vi "Main.vi"() -> ()   [LabVIEW 2021]
uses:
  Sub VIs/Trajectory Control/Trajectory_Control.ctl
  Sub VIs/Logging/Controller Data.ctl
  Sub VIs/Drive Motor/Drive Motor Data.ctl
  Sub VIs/Steering Motor/Steering Motor Data.ctl
  Sub VIs/State Estimator/State Estimate.ctl
  Sub VIs/State Estimator/Measurements.ctl
  Sub VIs/IMU/IMU Data.ctl
  Sub VIs/Steering Motor Encoder/Steering Motor Encoder Data.ctl
  Sub VIs/GNSS/GNSS Data.ctl
  <vilib>/Utility/RT CPU Load.ctl
  Sub VIs/Logging/Log Level.ctl
  <vilib>/Platform/TimedLoop/XDataNode/timing_clust.ctl
  <vilib>/Platform/TimedLoop/XDataNode/nitl_modes.ctl
  <vilib>/Platform/TimedLoop/XDataNode/wakeup.ctl
  Sub VIs/Steering Motor/Steering Motor Handle.ctl
  <vilib>/Platform/TimedLoop/XDataNode/XDataNode.xnode
  <vilib>/Platform/TimedLoop/XDataNode/XDNodeRunTimeDep.lvlib
  <vilib>/NI_Real-Time Target Support.lvlib
panel:
  in  "Abort Trajectory":bool
  in  "Kp":dbl
  in  "Ki":dbl
  out "Speed":bool
  in  "?":bool
  out "RPM":bool
  in  "Drive Motor Speed (m/s)":dbl
  in  "file path (trajectorymat)":path=path "c:/ni-rt/startup/trajectorymat_asta0_line.csv"
  in  "file path (matrixmat)":path=path "c:/ni-rt/startup/matrixmat_default.csv"
  out "velocity":dbl(graph)
  out "CPU loads":T1[](array[typedef]) {"ISR (%)" format="%#.2f"; "Idle (%)" format="%#.2f"; "Background (%)" format="%#.2f"; "Normal (%)" format="%#.2f"; "Above Normal (%)" format="%#.2f"; "High (%)" format="%#.2g"; "Timed Structures (%)" format="%#.2g"; "Time Critical (%)" format="%#.2g"; "Total (%)" format="%#.2g"}
  out "Measurements (Debug)":T2 {"GNSS Data"."Longitude (deg)" format="%#.10g"; "GNSS Data"."Latitude (deg)" format="%#.10g"; "GNSS Data"."Longitude (rad)" format="%#_10g"; "GNSS Data"."Latitude (rad)" format="%#_10g"}
  out "State Estimate (Debug)":T6 {"Y (m)" format="%#_10g"; "X (m)" format="%#_10g"}
  out "Motor Controllers (Debug)":T7
  out "Trajectory (Debug)":T10
  out "State estimator Ts check":bool
  out "E2 limit hit":bool
  out "E1 limit hit":bool
  out "XY trajectory (0 is bikeposition)":T11(graph)
  out "Y-Offset":dbl
  out "X-Offset":dbl
  in  "Reset and Init trajectory":bool
  in  "Drive Motor Angular Speed (rad/s)":dbl
  in  "Enable Steering Motor":bool
  out "Steering Motor Enabled":bool
  out "Abort":bool
  in  "Reset Steering Motor Encoder":bool
  in  "Stop Button":bool
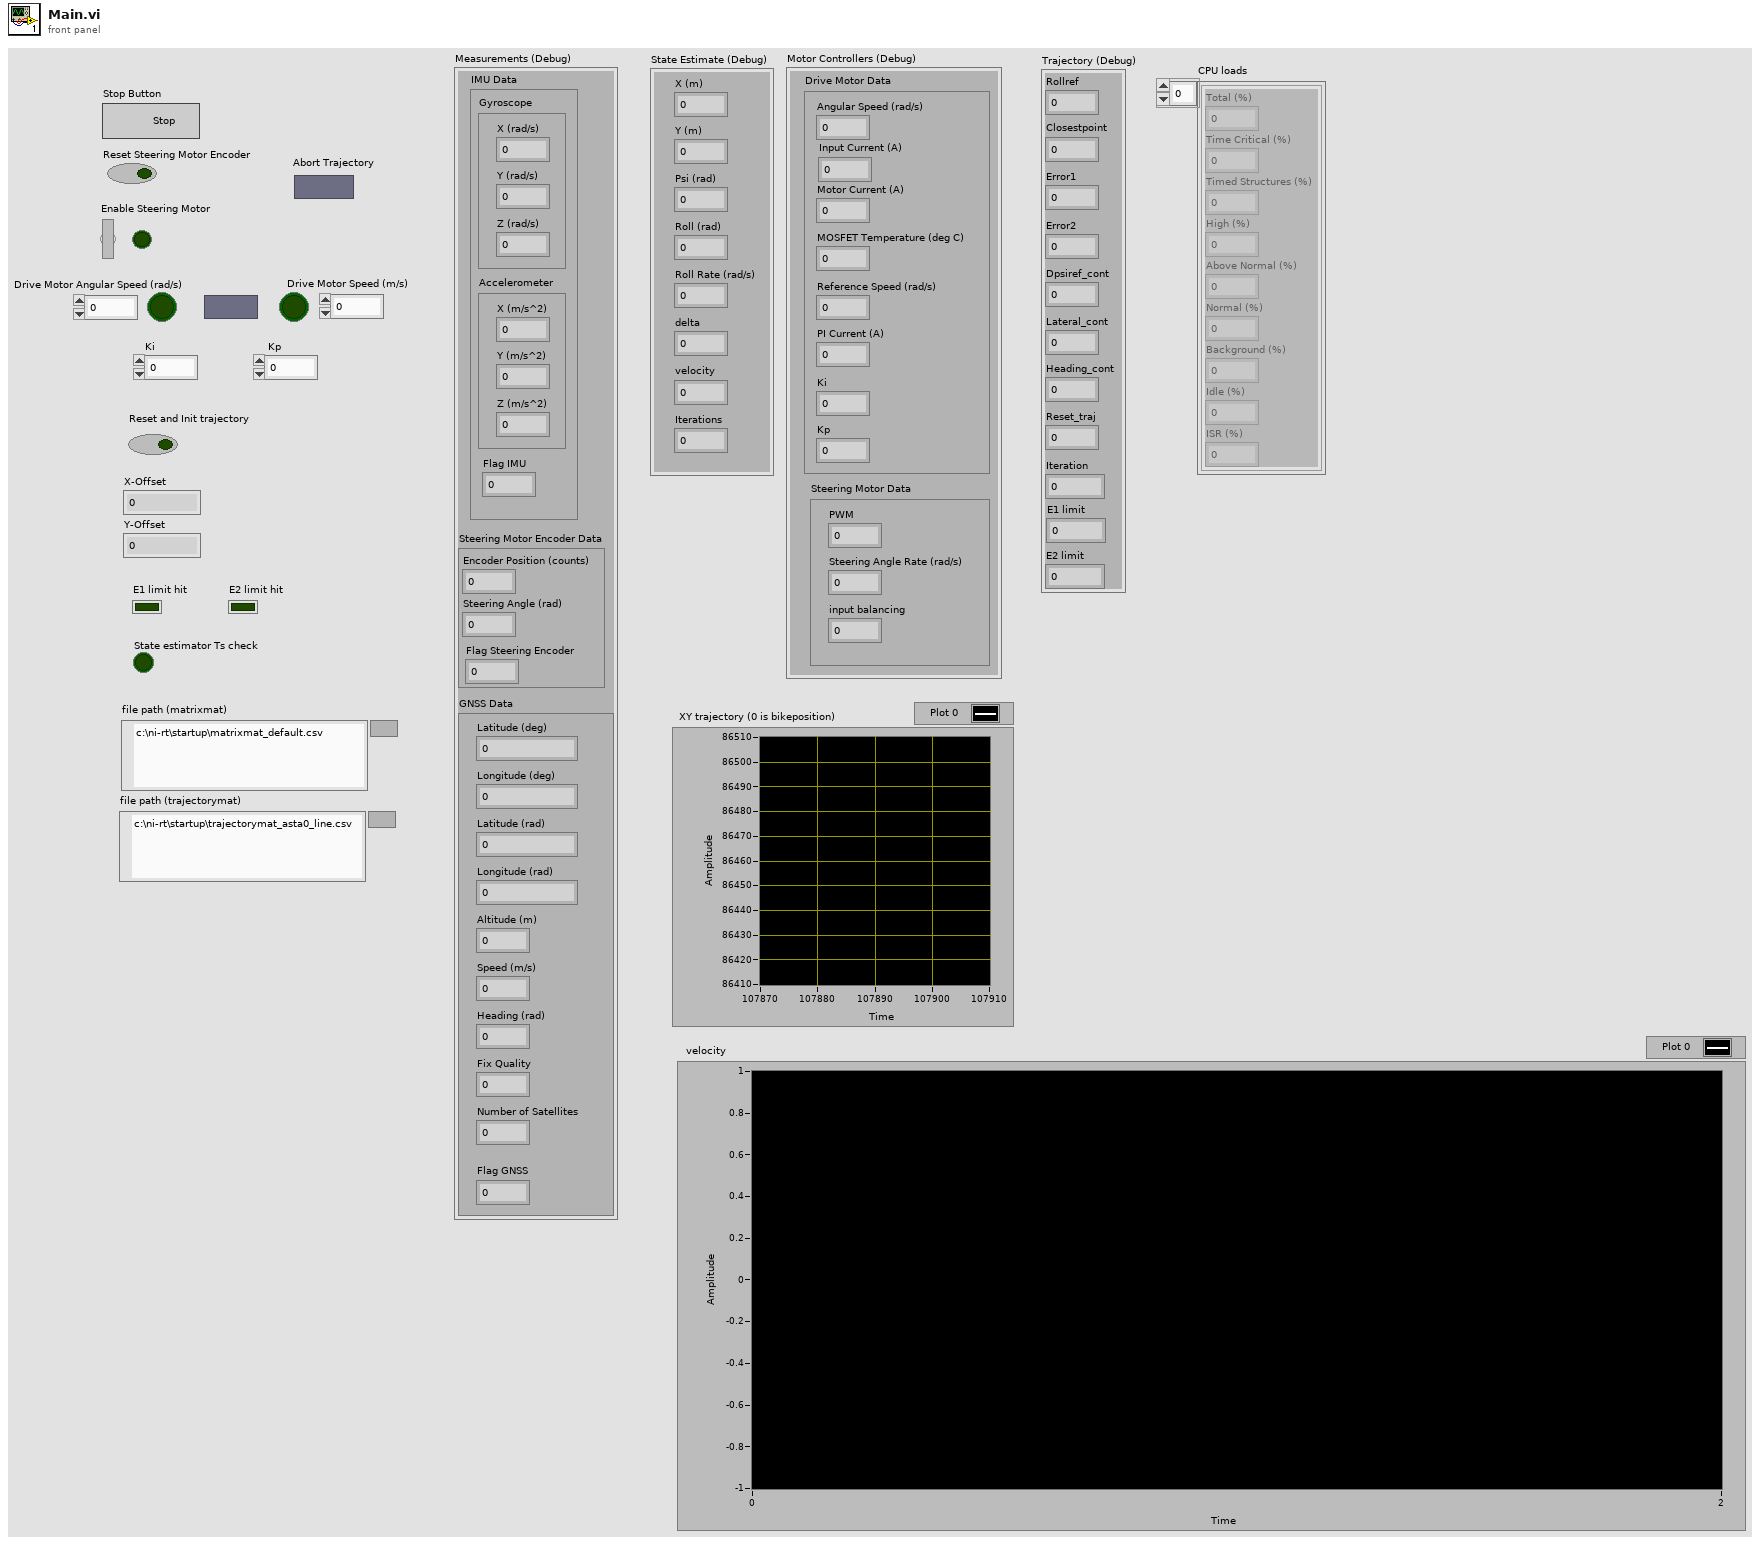
[diagram p1: front panel]
types:
  T1 = typedef "NI_Real-Time Target Support.lvlib/RT CPU Load.ctl" = cluster{"Total (%)":dbl, "Time Critical (%)":dbl, "Timed Structures (%)":dbl, "High (%)":dbl, "Above Normal (%)":dbl, "Normal (%)":dbl, "Background (%)":dbl, "Idle (%)":dbl, "ISR (%)":dbl}
  T2 = typedef "Measurements.ctl" = cluster{"IMU Data":T3, "Steering Motor Encoder Data":T4, "GNSS Data":T5}
  T3 = typedef "IMU Data.ctl" = cluster{"Gyroscope":cluster{"X (rad/s)":dbl, "Y (rad/s)":dbl, "Z (rad/s)":dbl}, "Accelerometer":cluster{"X (m/s^2)":dbl, "Y (m/s^2)":dbl, "Z (m/s^2)":dbl}, "Flag IMU":dbl}
  T4 = typedef "Steering Motor Encoder Data.ctl" = cluster{"Encoder Position (counts)":i32, "Steering Angle (rad)":dbl, "Flag Steering Encoder":dbl}
  T5 = typedef "GNSS Data.ctl" = cluster{"Latitude (rad)":dbl, "Longitude (rad)":dbl, "Altitude (m)":dbl, "Speed (m/s)":dbl, "Heading (rad)":dbl, "Fix Quality":i32, "Number of Satellites":i32, "Latitude (deg)":dbl, "Longitude (deg)":dbl, "Flag GNSS":dbl}
  T6 = typedef "State Estimate.ctl" = cluster{"X (m)":dbl, "Y (m)":dbl, "Psi (rad)":dbl, "Roll (rad)":dbl, "Roll Rate (rad/s)":dbl, "delta":dbl, "velocity":dbl, "Iterations":dbl}
  T7 = typedef "Controller Data.ctl" = cluster{"Drive Motor Data":T8, "Steering Motor Data":T9}
  T8 = typedef "Drive Motor Data.ctl" = cluster{"Angular Speed (rad/s)":dbl, "Input Current (A)":dbl, "Motor Current (A)":dbl, "MOSFET Temperature (deg C)":dbl, "Reference Speed (rad/s)":dbl, "PI Current (A)":dbl, "Ki":dbl, "Kp":dbl}
  T9 = typedef "Steering Motor Data.ctl" = cluster{"PWM":dbl, "Steering Angle Rate (rad/s)":dbl, "input balancing":dbl}
  T10 = typedef "Trajectory_Control.ctl" = cluster{"Rollref":dbl, "Closestpoint":dbl, "Error1":dbl, "Error2":dbl, "Dpsiref_cont":dbl, "Lateral_cont":dbl, "Heading_cont":dbl, "Reset_traj":dbl, "Iteration":dbl, "E1 limit":u32, "E2 limit":u32}
  T11 = cluster{"Trajectory(X/Y/PSI)":dbl[], "Trajectory(X/Y/PSI)":dbl[]}
  T12 = cluster{"Steering Angle Rate":dbl, "rollReference":dbl, "roll":dbl, "rollRate":dbl, "Kp":dbl, "Kd":dbl, "steering_flag":i32}
  T13 = typedef "XDNodeRunTimeDep.lvlib/timing_clust.ctl" = cluster{"Expected End [f-1]":u64, "Actual End [f-1]":u64, "Finished Late? [f-1]":bool, "Expected End [i-1]":u64, "Actual End [i-1]":u64, "Finished Late? [i-1]":bool, "Expected Start [i]":u64, "Actual Start [i]":u64, "Expected Start [f]":u64, "Actual Start [f]":u64, "Source Name":string, "Structure Name":string, "Period":i64, "Deadline":i64, "Offset":i64, "Start":i64, "Priority":i32, "Timeout":i32, "Mode":T14, "Wakeup Reason":T15, "Error":errorcluster, "Source Type":string, "Secondary Source Type":string, "Global End Time":u64, "Global Start Time":u64, "Frame Duration":u64, "Iteration Duration":u64, "Assigned CPU":i32, "I/O Scan Engine Mode":u32}
  T14 = typedef "XDNodeRunTimeDep.lvlib/nitl_modes.ctl" = enum32{"No Change", "Process missed periods, maintain original phase", "Discard missed periods, maintain original phase", "Process missed periods, ignore original phase", "Discard missed periods, ignore original phase"}
  T15 = typedef "XDNodeRunTimeDep.lvlib/wakeup.ctl" = enum32{"Normal", "Aborted", "Asynchronous wakeup", "Timing source error", "Timed loop error", "Timeout"}
  T16 = typedef "Steering Motor Handle.ctl" = cluster{"Dummy":dbl}
  T17 = typedef "Log Level.ctl" = enum16{"Error", "Warning", "Info"}
  T18 = cluster{"B":dbl[], "A":dbl[][], "C":dbl[][], "D":dbl[], "K":dbl[][], "Trajectory":dbl[][], "Init":dbl[], "parameter":dbl[][]}
  T19 = typedef "Configuration.ctl" = cluster{"Accelerometer Bias":cluster{"X (m/s)":dbl, "Y (m/s)":dbl, "Z (m/s)":dbl}, "Gyroscope Bias":cluster{"X (m/s)":dbl, "Y (m/s)":dbl, "Z (m/s)":dbl}, "Steering Motor Gear Ratio":dbl, "Steering Pully Gear Ratio":dbl, "Steering Encoder CPR":dbl, "Steering Motor Max RPM":dbl, "Wheelbase (m)":dbl, "Fork Angle (rad)":dbl, "Balancing Controller":cluster{"Kp (/s)":dbl, "Kd (1)":dbl}, "Max Allowed Steering Angle (rad)":dbl, "Task Periods":cluster{"Emergency Stop (us)":i64, "IMU (us)":i64, "Steering Motor Encoder (us)":i64, "State Estimator (us)":i64, "Balancing Controller (us)":i64, "GNSS (us)":i64, "Logging (us)":i64, "Drive Motor (us)":i64, "Visualization (us)":i64, "Reaction Wheel (us)":i64}, "Drive Motor Gear Ratio":dbl, "lr":dbl, "lf":dbl, "lambda":dbl, "k1":dbl, "k2":dbl, "e1_max":dbl, "Ad_t":dbl, "Bd_t":dbl, "C_t":dbl, "D_t":dbl, "Wheel radius":dbl}
  T20 = typedef "NI_Matrix.lvlib/RealMatrix.ctl" = dbl[][]
  T21 = typedef "IMU Handle.ctl" = cluster{"I2C address":u8}
  T22 = typedef "GNSS Handle.ctl" = cluster{"VISA Resource Name":refnum<visa-resource-name>}
  T23 = typedef "Drive Motor Handle.ctl" = cluster{"VISA Resource Name":refnum<visa-resource-name>}
  T24 = typedef "Log Handle.ctl" = cluster{"Data File":refnum<file>, "Event File":refnum<file>}
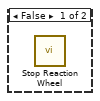
[diagram p2: hidden frame]
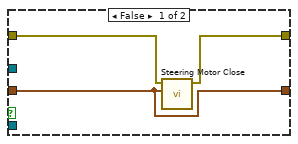
[diagram p4: hidden frame]
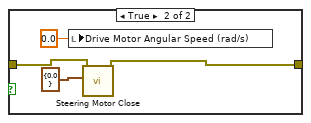
[diagram p5: hidden frame]
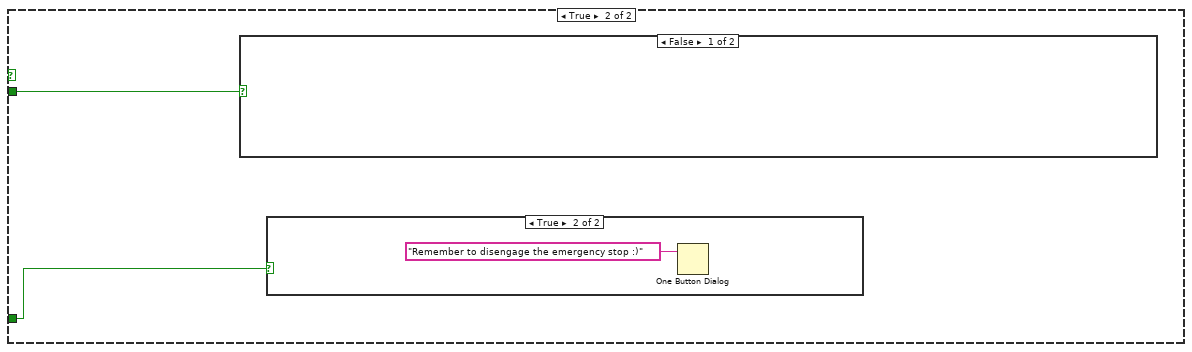
[diagram p6: hidden frame]
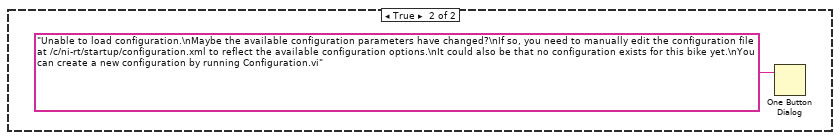
[diagram p7: hidden frame]
diagram:
  n1 = flat-sequence {
    frame #0 {
      n2 = call "Log Event.vi"("Clear Log"=TRUE) -> ()  [unwired: 10 in, 1 out]
    }
    frame #1 {
      n3 = call "Read Configuration.vi"("file path (trajectorymat)"="file path (trajectorymat)", "file path (matrixmat)"="file path (matrixmat)") -> ("values loded in xml files"=w9:T18, "configuration"=w11:T19, "value"=w4:T20, "error out"=w10:errorcluster, "Init trajectory (2)"=w6:dbl[][])  [unwired: 3 in, 2 out]
      n4 = call "Emergency Stop Read.vi"() -> ("Emergency Stop"=w7:bool)  [unwired: 10 in, 1 out]
      n5 = Unbundle By Name(w10) -> ("status"=w8:bool)
      n6 = Compound Arithmetic op=OR(w7, w8) -> (w5:bool)
      n7 = case shown="False" w5 {
        tunnel: w8 -> [_ w347]
        tunnel: w11 -> [w51 _]
        tunnel: w9 -> [w25 _]
        tunnel: w7 -> [_ w346]
        tunnel: w6 -> [w43 _]
        tunnel: w4 -> [w27 _]
        frame False {
          w33 = T10 {"Rollref"=0.0, "Closestpoint"=0.0, "Error1"=0.0, "Error2"=0.0, "Dpsiref_cont"=0.0, "Lateral_cont"=0.0, "Heading_cont"=0.0, "Reset_traj"=0.0, "Iteration"=0.0, "E1 limit"=0, "E2 limit"=0}  # Trajectory Init
          w44 = T6 {"X (m)"=0.0, "Y (m)"=0.0, "Psi (rad)"=0.0, "Roll (rad)"=0.0, "Roll Rate (rad/s)"=0.0, "delta"=0.0, "velocity"=0.0, "Iterations"=0.0}  # State Estimate Init
          w50 = T7 {"Drive Motor Data"={"Angular Speed (rad/s)"=0.0, "Input Current (A)"=0.0, "Motor Current (A)"=0.0, "MOSFET Temperature (deg C)"=0.0, "Reference Speed (rad/s)"=0.0, "PI Current (A)"=0.0, "Ki"=0.0, "Kp"=0.0}, "Steering Motor Data"={"PWM"=0.0, "Steering Angle Rate (rad/s)"=0.0, "input balancing"=0.0}}  # Motor controllers Init
          w73 = T2 {"IMU Data"={"Gyroscope"={"X (rad/s)"=0.0, "Y (rad/s)"=0.0, "Z (rad/s)"=0.0}, "Accelerometer"={"X (m/s^2)"=0.0, "Y (m/s^2)"=0.0, "Z (m/s^2)"=0.0}, "Flag IMU"=0.0}, "Steering Motor Encoder Data"={"Encoder Position (counts)"=0, "Steering Angle (rad)"=0.0, "Flag Steering Encoder"=0.0}, "GNSS Data"={"Latitude (rad)"=0.0, "Longitude (rad)"=0.0, "Altitude (m)"=0.0, "Speed (m/s)"=0.0, "Heading (rad)"=0.0, "Fix Quality"=0, "Number of Satellites"=0, "Latitude (deg)"=0.0, "Longitude (deg)"=0.0, "Flag GNSS"=0.0}}  # Measurements init
          n8 = flat-sequence {
            tunnel: [w342] -> w17
            tunnel: w51 -> [w342]
            frame #0 {
              n9 = invoke on="Stop Button" class="Bool (strict)" method="Reinit To Default"() -> ()  [unwired: 3 in, 3 out]
              n10 = local write "Abort"(FALSE ("Abort")) -> ()
              n11 = call "Log Event.vi"("Message"="Run started!", "Log Level"=Log_Level."Info") -> ()  [unwired: 9 in, 1 out]
            }
          }
          n12 = Unbundle By Name(w17) -> ("Task Periods.Emergency Stop (us)"=w72:i64)
          n13 = node-c288(w72) -> (w71:T13)
          n14 = timed-loop {
            timing: w71 -> [_]
            timing-out: [_] -> w70
            stop <- w325 stop-if-true
            # "Emergency Stop"
            n15 = node-c288() -> (w327:errorcluster)  [unwired: 1 in]
            n16 = call "Emergency Stop Read.vi"("Error In"=w327) -> ("Emergency Stop"=w322:bool, "Error Out"=w323:errorcluster)  [unwired: 9 in]
            n17 = Or(x=w322, y="Stop Button") -> (x .or. y?=w325:bool)
            "Abort" <- w325
            n18 = case shown="False" w325 {
              tunnel: w327 -> [_ w332]
              tunnel: [errorcluster {"status"=FALSE, "code"=0, "source"=""} ("Error Out") w331] -> w324
              frame False {
              }
              frame True {
                n19 = local write "Drive Motor Angular Speed (rad/s)"(0.0 ("Drive Motor Angular Speed (rad/s)")) -> ()
                n20 = call "Steering Motor Close.vi"("Steering Motor Handle"=T16 {"Dummy"=0.0}, "Error In"=w332) -> ("Error Out"=w331:errorcluster)  [unwired: 9 in]
              }
            }
            n21 = Merge Errors(w324, w323) -> (w326:errorcluster)
            n22 = node-c288(w326) -> ()  [unwired: 1 out]
          }
          n23 = node-c288(w70) -> ()  [unwired: 1 out]
          n24 = New Data Value Reference(data value=w73) -> (data value reference=w21:refnum<data-value>)  [unwired: 1 in, 1 out]
          n25 = Unbundle By Name(w17) -> ("Task Periods.Steering Motor Encoder (us)"=w56:i64)
          n26 = Unbundle By Name(w17) -> ("Task Periods.GNSS (us)"=w53:i64)
          n27 = Unbundle By Name(w17) -> ("Task Periods.IMU (us)"=w57:i64)
          n28 = call "IMU Configure.vi"() -> ("IMU Handle"=w58:T21, "Error Out"=w59:errorcluster)  [unwired: 10 in]
          n29 = call "GNSS Open.vi"() -> ("GNSS Handle"=w54:T22, "Error Out"=w55:errorcluster)  [unwired: 10 in]
          n30 = node-c288(w56) -> (w63:T13)
          n31 = node-c288(w57, w59) -> (w65:T13)
          n32 = node-c288(w53, w55) -> (w61:T13)
          n33 = timed-loop {
            timing: w63 -> [_]
            timing-out: [_] -> w62
            tunnel: w21 -> [w244]
            tunnel: w17 -> [w242]
            i -> [w243]
            stop <- w245 stop-if-true
            # "Steering Motor Encoder"
            n34 = node-c288() -> (w248:errorcluster)  [unwired: 1 in]
            n35 = call "Steering Motor Encoder Read.vi"("Configuration"=w242, "Measurement In"=w244, "Flag Steering Encoder"=w243, "Reset Counter"="Reset Steering Motor Encoder", "Error In"=w248) -> ("Error Out"=w247:errorcluster)  [unwired: 4 in, 2 out]
            n36 = local read "Abort"() -> (w245:bool)
            n37 = node-c288(w247) -> ()  [unwired: 1 out]
          }
          n38 = timed-loop {
            timing: w65 -> [_]
            timing-out: [_] -> w64
            tunnel: w58 -> [w262]
            tunnel: w21 -> [w260]
            tunnel: w17 -> [w259]
            i -> [w258]
            stop <- w261 stop-if-true
            # "IMU"
            n39 = node-c288() -> (w264:errorcluster)  [unwired: 1 in]
            n40 = call "IMU Read.vi"("Configuration"=w259, "Measurement In"=w260, "Flag IMU"=w258, "IMU Handle"=w262, "Error In"=w264) -> ("Error Out"=w263:errorcluster)  [unwired: 4 in, 2 out]
            n41 = local read "Abort"() -> (w261:bool)
            n42 = node-c288(w263) -> ()  [unwired: 1 out]
          }
          n43 = timed-loop {
            timing: w61 -> [_]
            timing-out: [_] -> w60
            tunnel: w54 -> [w231]
            tunnel: w21 -> [w227]
            tunnel: [w225] -> _
            stop <- w228 stop-if-true
            # "GNSS"
            n44 = node-c288() -> (w230:errorcluster)  [unwired: 1 in]
            n45 = call "GNSS Read.vi"("Measurement In"=w227, "GNSS Handle"=w231, "Error In"=w230) -> ("GNSS Data"=w226:T5, "Error Out"=w229:errorcluster)  [unwired: 6 in, 1 out]
            n46 = Unbundle By Name(w226) -> ("Speed (m/s)"=w225:dbl)
            "velocity" <- w225
            n47 = local read "Abort"() -> (w228:bool)
            n48 = node-c288(w229) -> ()  [unwired: 1 out]
          }
          n49 = node-c288(w62) -> ()
          n50 = node-c288(w64) -> ()
          n51 = Unbundle By Name(w25) -> ("Trajectory"=w32:dbl[][])
          n52 = New Data Value Reference(data value=w32) -> (data value reference=w26:refnum<data-value>)  [unwired: 1 in, 1 out]
          n53 = node-c288(w60) -> ()
          n54 = New Data Value Reference(data value=w33) -> (data value reference=w15:refnum<data-value>)  [unwired: 1 in, 1 out]
          n55 = New Data Value Reference(data value=w44) -> (data value reference=w16:refnum<data-value>)  [unwired: 1 in, 1 out]
          n56 = New Data Value Reference(data value=w50) -> (data value reference=w22:refnum<data-value>)  [unwired: 1 in, 1 out]
          n57 = disable-structure shown="Disabled" {
            disable-tunnel: w26 -> [w100 _]
            disable-tunnel: w21 -> [w99 _]
            disable-tunnel: w17 -> [w98 _]
            disable-tunnel: w16 -> [w97 _]
            disable-tunnel: w15 -> [w96 _]
            frame Disabled {
              n58 = Unbundle By Name(w98) -> ("Task Periods.State Estimator (us)"=w101:i64)
              n59 = node-c288(w101) -> (w103:T13)
              n60 = timed-loop {
                timing: w103 -> [_]
                timing-out: [_] -> w102
                tunnel: w97 -> [w115]
                tunnel: w98 -> [w112]
                tunnel: w99 -> [w110]
                tunnel: w100 -> [w109]
                tunnel: w96 -> [w107]
                i -> [w111]
                stop <- w116 stop-if-true
                # "Trajectory controller"
                n61 = node-c288() -> (w113:errorcluster)  [unwired: 1 in, 1 out]
                n62 = call "Trajectory_Controller.vi"("Error In"=w113, "reset"=w111, "Abort Trajectory"="Abort Trajectory", "Configuration"=w112, "State Estimate In"=w115, "Reset and Init trajectory"="Reset and Init trajectory", "RefTraj in"=w109, "Trajectory In"=w107, "Measurement In"=w110) -> ("Error out"=w114:errorcluster, "E1 limit"=→"E1 limit hit":bool, "E2 limit"=→"E2 limit hit":bool)  [unwired: 2 in, 2 out]
                n63 = local read "Abort"() -> (w116:bool)
                n64 = node-c288(w114) -> ()  [unwired: 1 out]
              }
              n65 = node-c288(w102) -> ()
            }
            frame Enabled {
            }
          }
          n66 = Unbundle By Name(w17) -> ("Task Periods.State Estimator (us)"=w23:i64)
          n67 = Unbundle By Name(w17) -> ("Task Periods.Reaction Wheel (us)"=w12:i64)
          n68 = Unbundle By Name(w17) -> ("Task Periods.Visualization (us)"=w28:i64)
          n69 = node-c288(w23) -> (w35:T13)
          n70 = node-c288(w12) -> (w14:T13)
          n71 = timed-loop {
            timing: w35 -> [_]
            timing-out: [_] -> w34
            tunnel: w21 -> [w159]
            tunnel: w25 -> [w162]
            tunnel: w22 -> [w158]
            tunnel: w16 -> [w157]
            tunnel: w17 -> [w161]
            i -> [w160]
            stop <- w165 stop-if-true
            w151 = i64 12 ("y")
            # "State Estimator kalman"
            n72 = node-c288() -> (w164:errorcluster)  [unwired: 1 in]
            n73 = call "State Estimator.vi"("Error In"=w164, "State Estimate In"=w157, "Matrix"=w162, "Configuration"=w161, "Iteration"=w160, "Measurement In"=w159, "Balancing controller In"=w158) -> ("Error out"=w163:errorcluster)  [unwired: 7 in, 1 out]
            n74 = Tick Count (ms)() -> (millisecond timer value=w156:u32)
            n75 = feedback-in #1(w156) -> ()
            n76 = feedback #1() -> (w155:u32)  [unwired: 1 in]
            n77 = Negate(x=w151) -> (-x=w152:i64)
            n78 = Subtract(x=w156, y=w155) -> (x-y=w153:u32)
            n79 = local read "Abort"() -> (w165:bool)
            n80 = In Range and Coerce(upper limit=w151, x=w153, lower limit=w152) -> (In Range?=→"State estimator Ts check":bool)  [unwired: 1 out]
            n81 = node-c288(w163) -> ()  [unwired: 1 out]
          }
          n82 = timed-loop {
            timing: w14 -> [_]
            timing-out: [_] -> w13
            tunnel: w16 -> [w84]
            tunnel: w15 -> [w77]
            stop <- _ stop-if-true
            w81 = 0
            # "Suggestion for integration into Autobike code. Define some velocity range where reaction wheel should be active."
            n83 = node-c288() -> ()  [unwired: 1 in, 1 out]
            n84 = in-place {
              in-place-border: [w89] -> w83
              n85 = in-place-dvr #2(w84) -> (w89:T6)  [unwired: 1 out]
              n86 = in-place-dvr #2(w89) -> ()  [unwired: 2 out]
            }
            n87 = in-place {
              in-place-border: [w88] -> w76
              n88 = in-place-dvr #3(w77) -> (w88:T10)  [unwired: 1 out]
              n89 = in-place-dvr #3(w88) -> ()  [unwired: 2 out]
            }
            n90 = Unbundle By Name(w83) -> ("velocity"=w82:dbl, "Roll (rad)"=w75:dbl)
            n91 = In Range and Coerce(upper limit=w81, x=w82, lower limit=w81) -> (In Range?=w79:bool)  [unwired: 1 out]
            n92 = local read "Abort"() -> (w80:bool)
            n93 = Not(x=w79) -> (.not. x?=w78:bool)
            n94 = Or(x=w80, y=w78) -> (x .or. y?=w74:bool)
            n95 = case shown="True" w74 {
              tunnel: w76 -> [_ w87]
              tunnel: w75 -> [_ w85]
              frame False {
                n96 = call "Stop Reaction Wheel.vi"() -> ()  [unwired: 12 in]
              }
              frame True {
                n97 = Unbundle By Name(w87) -> ("Rollref"=w86:dbl)
                n98 = call "SubVI ReactionWheel.vi"("Roll angle"=w85, "Roll reference"=w86) -> ()  [unwired: 9 in, 1 out]
              }
            }
            n99 = node-c288() -> ()  [unwired: 1 in, 1 out]
          }
          n100 = node-c288(w34) -> ()
          n101 = node-c288(w13) -> ()  [unwired: 1 out]
          n102 = flat-sequence {
            tunnel: [w276] -> w52
            tunnel: w17 -> [w275]
            frame #0 {
              n103 = Unbundle By Name(w275) -> ("Task Periods.Balancing Controller (us)"=w276:i64)
              n104 = local write "Enable Steering Motor"(FALSE ("Enable Steering Motor")) -> ()
            }
          }
          n105 = New Data Value Reference(data value=T12 {"Steering Angle Rate"=0.0, "rollReference"=0.0, "roll"=0.0, "rollRate"=0.0, "Kp"=0.0, "Kd"=0.0, "steering_flag"=0} ("output cluster")) -> (data value reference=w19:refnum<data-value>)  [unwired: 1 in, 1 out]
          n106 = Unbundle By Name(w17) -> ("Task Periods.Drive Motor (us)"=w18:i64)
          n107 = call "Drive Motor Init.vi"() -> ("Drive Motor Handle"=w40:T23, "Error Out"=w39:errorcluster)  [unwired: 10 in]
          n108 = node-c288(w18, w39) -> (w42:T13)
          n109 = timed-loop {
            timing: w42 -> [_]
            timing-out: [_] -> w41
            tunnel: w40 -> [w187]
            tunnel: w17 -> [w183]
            tunnel: w22 -> [w184]
            tunnel: [w188] -> w36
            tunnel: w18 -> [w175]
            stop <- w189 stop-if-true
            # "Drive Controller"
            n110 = node-c288() -> (w186:errorcluster)  [unwired: 1 in]
            n111 = Not(x="?") -> (.not. x?=→"RPM":bool)
            n112 = To Single Precision Float(number=w175) -> (single precision float=w176:sgl)
            n113 = call "Drive Motor TXRX.vi"("Error In"=w186, "Speed Control (m/s)"="Drive Motor Speed (m/s)", "RPM / Speed"="?", "Drive Motor Handle In"=w187, "Tasking Period"=w176, "RPM Control (rad/s)"="Drive Motor Angular Speed (rad/s)", "Controller Data In"=w184, 12:w183, "Ki"="Ki", "Kp"="Kp") -> ("Error Out"=w185:errorcluster, "Drive Motor Handle Out"=w188:T23)  [unwired: 2 in, 2 out]
            n114 = local read "Abort"() -> (w189:bool)
            n115 = node-c288(w185) -> ()  [unwired: 1 out]
            "Speed" <- "?"
          }
          n116 = node-c288(w52) -> (w69:T13)
          n117 = timed-loop {
            timing: w69 -> [_]
            timing-out: [_] -> w68
            tunnel: w16 -> [w287]
            tunnel: w21 -> [w286]
            shift-right: [w288] -> w67
            shift-left: _ -> [w285]
            tunnel: w17 -> [w284]
            tunnel: w22 -> [w283]
            tunnel: w15 -> [w282]
            tunnel: w19 -> [w279]
            i -> [w278]
            stop <- w291 stop-if-true
            # "Balancing Controller"
            n118 = node-c288() -> (w290:errorcluster)  [unwired: 1 in]
            n119 = Boolean To (0,1)(Boolean="Enable Steering Motor") -> (0, 1=w280:i16)
            n120 = case shown="True" "Enable Steering Motor" {
              tunnel: w290 -> [w294 w304]
              tunnel: [w293 w309] -> w289
              tunnel: [w292 w308] -> w288
              tunnel: w287 -> [_ w306]
              tunnel: w286 -> [_ w305]
              tunnel: w285 -> [w292 _]
              tunnel: w284 -> [_ w300]
              tunnel: w283 -> [_ w301]
              tunnel: w282 -> [_ w299]
              tunnel: w280 -> [_ w297]
              tunnel: w279 -> [_ w296]
              tunnel: w278 -> [_ w295]
              frame False {
                n121 = call "Steering Motor Close.vi"("Steering Motor Handle"=w292, "Error In"=w294) -> ("Error Out"=w293:errorcluster)  [unwired: 9 in]
              }
              frame True {
                n122 = call "Steering Motor Open.vi"("Error In"=w304) -> ("Steering Motor Handle"=w302:T16, "Error Out"=w303:errorcluster)  [unwired: 9 in]
                n123 = call "Balancing Controller.vi"("t"=w295, "Balance In"=w296, "Configuration"=w300, "steering indicator flag"=w297, "Measurement In"=w305, "State Estimate In"=w306, "Trajectory In"=w299, "Error In"=w303) -> ("Error Out"=w310:errorcluster, "Steering Angle Rate (rad/s)"=w307:dbl, "Input balancing"=w298:dbl)  [unwired: 1 out]
                n124 = call "Steering Motor Write.vi"("Configuration"=w300, "Input balancing"=w298, "Controller Data In"=w301, "Steering Angle Rate (rad/s)"=w307, "Steering Motor Handle In"=w302, "Error In"=w310) -> ("Steering Motor Handle Out"=w308:T16, "Error Out"=w309:errorcluster)  [unwired: 2 in, 2 out]
              }
            }
            n125 = local read "Abort"() -> (w291:bool)
            n126 = node-c288(w289) -> ()  [unwired: 1 out]
            "Steering Motor Enabled" <- "Enable Steering Motor"
          }
          n127 = node-c288(w41) -> (w38:errorcluster)
          n128 = node-c288(w68) -> (w66:errorcluster)
          n129 = call "Drive Motor TXRX.vi"("Error In"=w38, "Drive Motor Handle In"=w36, "RPM Control (rad/s)"=0.0 ("Angular Speed (rad/s)"), "Controller Data In"=w22, 12:w17) -> ()  [unwired: 7 in, 4 out]
          n130 = call "Steering Motor Close.vi"("Steering Motor Handle"=w67, "Error In"=w66) -> ()  [unwired: 9 in, 1 out]
          n131 = Unbundle By Name(w17) -> ("Task Periods.Logging (us)"=w24:i64)
          n132 = call "Log Init.vi"("Configuration"=w17, "Matrices"=w27, "Trajectory"=w43) -> ("Log Handle"=w45:T24, "Error Out"=w47:errorcluster)  [unwired: 7 in]
          n133 = node-c288(w28) -> (w30:T13)
          n134 = node-c288(w24, w47) -> (w49:T13)
          n135 = timed-loop {
            timing: w30 -> [_]
            timing-out: [_] -> w29
            tunnel: w26 -> [w136]
            tunnel: w21 -> [w135]
            tunnel: w22 -> [w131]
            tunnel: w21 -> [w130]
            tunnel: w16 -> [w129]
            tunnel: w15 -> [w128]
            stop <- w126 stop-if-true
            # "Visualization and Position Check"
            n136 = node-c288() -> (w137:errorcluster)  [unwired: 1 in]
            n137 = call <vilib>:"RT Get CPU Loads.vi"() -> ("CPU loads"=→"CPU loads":T1[])  [unwired: 10 in, 1 out]
            n138 = in-place {
              n139 = in-place-dvr #4(w128) -> (w138:T10)  [unwired: 1 out]
              "Trajectory (Debug)" <- w138
              n140 = in-place-dvr #4(w138) -> ()  [unwired: 2 out]
            }
            n141 = in-place {
              n142 = in-place-dvr #5(w131) -> (w139:T7)  [unwired: 1 out]
              "Motor Controllers (Debug)" <- w139
              n143 = in-place-dvr #5(w139) -> ()  [unwired: 2 out]
            }
            n144 = call "Position Check.vi"("data value reference 2"=w135, "data value reference"=w136) -> ("Y-Offset"=→"Y-Offset":dbl, "X-Offset"=→"X-Offset":dbl, "XY Graph"=→"XY trajectory (0 is bikeposition)":T11)  [unwired: 7 in]
            n145 = in-place {
              n146 = in-place-dvr #6(w130) -> (w141:T2)  [unwired: 1 out]
              "Measurements (Debug)" <- w141
              n147 = in-place-dvr #6(w141) -> ()  [unwired: 2 out]
            }
            n148 = in-place {
              n149 = in-place-dvr #7(w129) -> (w140:T6)  [unwired: 1 out]
              "State Estimate (Debug)" <- w140
              n150 = in-place-dvr #7(w140) -> ()  [unwired: 2 out]
            }
            n151 = local read "Abort"() -> (w126:bool)
            n152 = node-c288(w137) -> ()  [unwired: 1 out]
          }
          n153 = timed-loop {
            timing: w49 -> [_]
            timing-out: [_] -> w48
            tunnel: w21 -> [w203]
            tunnel: w16 -> [w206]
            shift-right: [w208] -> w31
            shift-left: w45 -> [w207]
            tunnel: w22 -> [w205]
            tunnel: w15 -> [w204]
            tunnel: w15 -> [_]
            tunnel: w19 -> [w201]
            i -> [w202]
            stop <- w213 stop-if-true
            # "Logging"
            n154 = node-c288() -> (w210:errorcluster)  [unwired: 1 in]
            n155 = Equal?(x=w202, y=0) -> (x = y?=w211:bool)
            n156 = call "Log Write.vi"("Error In"=w210, "Write Header"=w211, "Log Handle In"=w207, "Trajectory In"=w204, "State Estimate In"=w206, "Measurement In"=w203, "Controller Data In"=w205, "Balance In"=w201) -> ("Error Out"=w209:errorcluster, "Log Handle Out"=w208:T24)  [unwired: 1 in, 5 out]
            n157 = node-c288(w209) -> ()  [unwired: 1 out]
            n158 = local read "Abort"() -> (w213:bool)
          }
          n159 = node-c288(w48) -> (w46:errorcluster)
          n160 = call "Log Close.vi"("Log Handle In"=w31, "Error In"=w46) -> ()  [unwired: 9 in, 1 out]
          n161 = node-c288(w29) -> ()
        }
        frame True {
          n162 = case shown="False" w347 {
            frame False {
            }
            frame True {
              n163 = One Button Dialog(message="Unable to load configuration.\nMaybe the available configuration parameters have changed?\nIf so, you need to manually edit the configuration file at /c/ni-rt/startup/configuration.xml to reflect the available configuration options.\nIt could also be that no configuration exists for this bike yet.\nYou can create a new configuration by running Configuration.vi") -> ()  [unwired: 1 in, 1 out]
            }
          }
          n164 = case shown="True" w346 {
            frame False {
            }
            frame True {
              n165 = One Button Dialog(message="Remember to disengage the emergency stop :)") -> ()  [unwired: 1 in, 1 out]
            }
          }
        }
      }
    }
  }
